vi "REWORK_alternate_colors_by_timestamp_difference.vi"(6 "message_history_buffer":T1[](array[typedef]), 8 "error_in":errorcluster, 11 "listbox_ref":refnum<vi>) -> (0 "error_out":errorcluster)   [LabVIEW 2019]
uses:
  FGV/DIAGNOSTICS_message_history_buffer/REWORK_DIAGNOSTICS_message_history_buffer_all_info.ctl
  _misc/DIAGNOSTICS_message_type.ctl
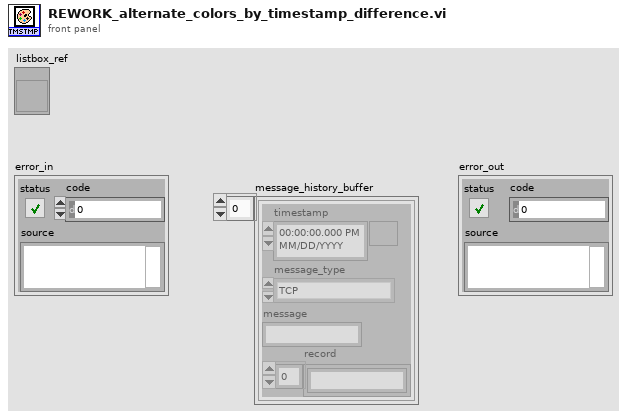
[diagram p1: front panel]
types:
  T1 = typedef "REWORK_DIAGNOSTICS_message_history_buffer_all_info.ctl" = cluster{"timestamp":timestamp, "message_type":T2, "message":string, "record":string[]}
  T2 = typedef "DIAGNOSTICS_message_type.ctl" = enum16{"TCP", "SQL"}
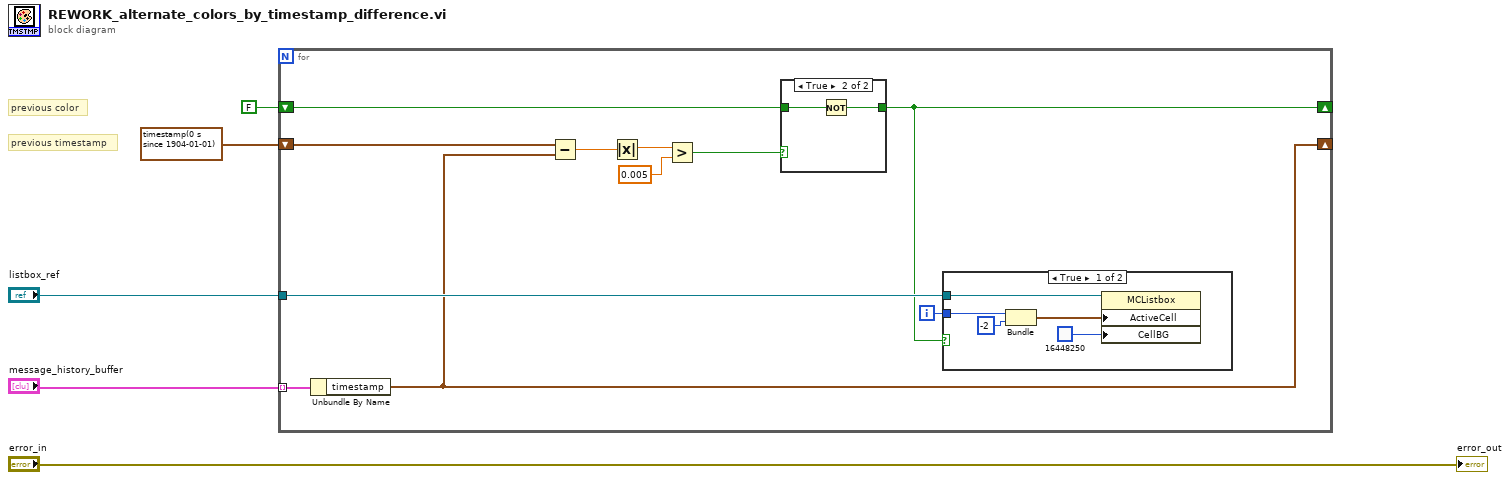
[diagram p0: block diagram]
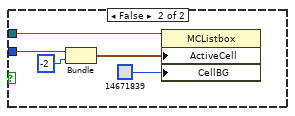
[diagram p3: hidden frame]
diagram:
  # "previous timestamp"
  # "previous color"
  n1 = for {
    tunnel: "listbox_ref" -> [w16]
    tunnel: "message_history_buffer" -> [w14] mode=indexing
    shift-right: [w7] -> _
    shift-left: FALSE -> [w10]
    shift-right: [w8] -> _
    shift-left: timestamp(0 s since 1904-01-01) ("timestamp") -> [w9]
    i -> [w15]
    n2 = Unbundle By Name(w14) -> ("timestamp"=w8:timestamp)
    n3 = Subtract(x=w9, y=w8) -> (x-y=w13:dbl)
    n4 = Absolute Value(x=w13) -> (abs(x)=w12:dbl)
    n5 = Greater?(x=w12, y=0.005) -> (0:w6:bool)
    n6 = case shown="True" w6 {
      tunnel: w10 -> [w17 w19]
      tunnel: [w17 w18] -> w7
      frame False {
      }
      frame True {
        n7 = Not(x=w19) -> (.not. x?=w18:bool)
      }
    }
    n8 = case shown="True" w7 {
      tunnel: w16 -> [w20 w29]
      tunnel: w15 -> [w21 w25]
      frame True {
        n9 = Bundle(w21, -2) -> (w23:cluster{i32, i32})  [unwired: 1 in]
        n10 = property on="Property Node" class="MCListbox"(reference=w20, "ActiveCell"=w23, "CellBG"=u32 16448250) -> ()  [unwired: 1 in, 2 out]
      }
      frame False {
        n11 = Bundle(w25, -2) -> (w27:cluster{i32, i32})  [unwired: 1 in]
        n12 = property on="Property Node" class="MCListbox"(reference=w29, "ActiveCell"=w27, "CellBG"=u32 14671839) -> ()  [unwired: 1 in, 2 out]
      }
    }
  }
  "error_out" <- "error_in"
